vi "GetBoolean.vi"(6 "false string (0)":string="0", 7 "key description":string, 8 "sections":string[](array[string]), 9 "boolean":bool, 11 "info data":string) -> (0 "sections out":string[](array[string]), 2 "value":bool, 3 "info data out":string)   [LabVIEW 2019, in "infolib.lvlib"]
doc: "Add a new numeric key to Info Data string. If section exists in Info Data string, inserts key into this section."
uses:
  infolib.lvlib
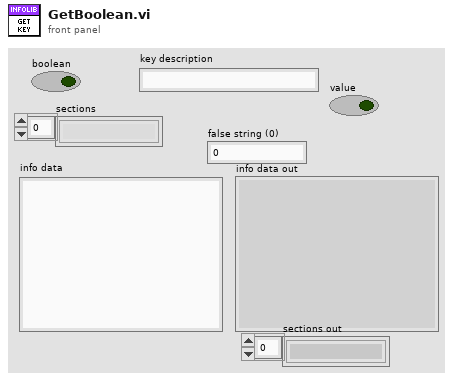
[diagram p1: front panel]
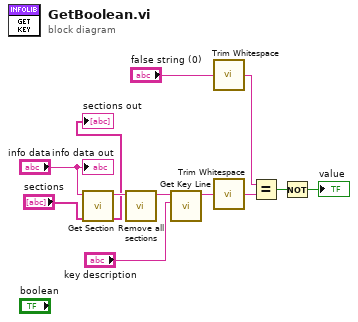
[diagram p0: block diagram]
diagram:
  n1 = call "Get Section.vi"("sections"="sections", "info data"="info data") -> ("sections out"=→"sections out":string[], "section part"=w12:string)  [unwired: 7 in, 1 out]
  n2 = call "Remove all sections.vi"("info data"=w12) -> ("info data out"=w11:string)  [unwired: 10 in]
  n3 = call "Get Key Line.vi"("key description"="key description", "info data"=w11) -> ("key value"=w5:string)  [unwired: 9 in]
  n4 = call <vilib>:"Trim Whitespace.vi"("string"="false string (0)") -> ("trimmed string"=w7:string)  [unwired: 1 in]
  n5 = call <vilib>:"Trim Whitespace.vi"("string"=w5) -> ("trimmed string"=w6:string)  [unwired: 1 in]
  n6 = Equal?(x=w7, y=w6) -> (x = y?=w4:bool)
  n7 = Not(x=w4) -> (.not. x?=→"value":bool)
  "info data out" <- "info data"
